vi "CRYArray replace with extend.vi"(7 "Enable (T)":bool=TRUE, 9 "Index":i32, 10 "String element":string, 11 "String array":string[](array[string])) -> (3 "String array out":string[](array[string]))   [LabVIEW 2013]
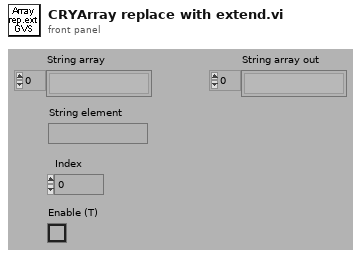
[diagram p1: front panel]
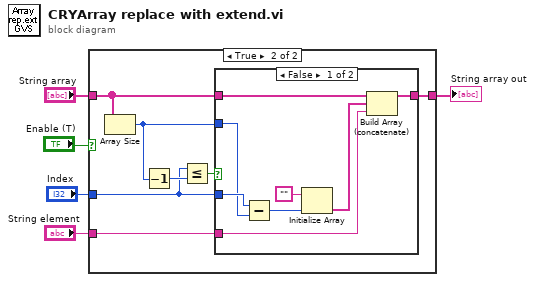
[diagram p0: block diagram]
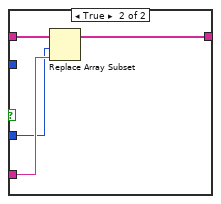
[diagram p3: hidden frame]
diagram:
  n1 = case shown="True" "Enable (T)" {
    tunnel: "String array" -> [w6 w11]
    tunnel: "String element" -> [_ w10]
    tunnel: "Index" -> [_ w9]
    tunnel: [w6 w8] -> w2
    frame False {
    }
    frame True {
      n2 = Array Size(array=w11) -> (size(s)=w7:i32)
      n3 = Decrement(x=w7) -> (x-1=w13:i32)
      n4 = Less Or Equal?(x=w9, y=w13) -> (x <= y?=w12:bool)
      n5 = case shown="False" w12 {
        tunnel: w11 -> [w17 w25]
        tunnel: w10 -> [w15 w24]
        tunnel: w9 -> [w21 w23]
        tunnel: [w14 w22] -> w8
        tunnel: w7 -> [w20 _]
        frame False {
          n6 = Subtract(x=w21, y=w20) -> (x-y=w19:i32)
          n7 = Initialize Array("", w19) -> (w16:string[])
          n8 = Build Array (concatenate)(w17, w16, w15) -> (w14:string[])
        }
        frame True {
          n9 = Replace Array Subset(array=w25, new element=w24, index=w23) -> (w22:string[])
        }
      }
    }
  }
  "String array out" <- w2
